vi "Actor Core.vi"(8 "error in":errorcluster, 11 "IViewable In":refnum<class "IViewable.lvclass">) -> (0 "error out":errorcluster, 3 "Actor out":refnum<class "Actor.lvclass">)   [LabVIEW 2017, in "IViewable.lvlib" / "IViewable.lvclass"]
doc: "(<B>Filename</B>: Actor Framework.lvlib:Actor.lvclass:Actor Core.vi)\n\nReceives messages to the actor, reacts to them, and initiates any error handling that may shut the actor down.\n\nDescendant classes may override this VI to append parallel tasks for the actor to complete while it handles messages. Overrides use the Call Parent Method node.\n\n<License>\nCopyright © 2017 Composed Systems, LLC | All rights reserved\nwww.composed.io\n\nAuthor: Ethan Stern <ethan.stern@composed.io>\n\nThis software is provided \"AS IS\" WITHOUT WARRANTIES, either express or implied, AND IS FOR EDUCATIONAL PURPOSES ONLY.\n</License>"
uses:
  IViewable.lvclass
  C:/Program Files (x86)/National Instruments/LabVIEW 2017/vi.lib/ActorFramework/Actor/Actor.lvclass
  <vilib>/ActorFramework/Actor/Actor.lvclass
  IViewable.lvclass/IViewable.ctl
  <vilib>/ActorFramework/Actor/Actor.lvclass/Actor.ctl
  <vilib>/ActorFramework/Message Enqueuer/Message Enqueuer.lvclass/Message Enqueuer.ctl
  IViewable Messages/Resize Panel to Pane Msg/Resize Panel to Pane Msg.lvclass/Resize Panel to Pane Msg.ctl
  <vilib>/ActorFramework/Message Enqueuer/Init from Existing Queue.vi
  <vilib>/ActorFramework/Message Enqueuer/Enqueue.vi
  IViewable Messages/Resize Panel to Pane Msg/Resize Panel to Pane Msg.lvclass
  C:/Program Files (x86)/National Instruments/LabVIEW 2017/vi.lib/ActorFramework/Message/Message.lvclass
  <vilib>/ActorFramework/Message Priority Queue/Priority Enqueue.vi
  <vilib>/ActorFramework/Message Enqueuer/Message Enqueuer.lvclass
  ActorEvents/IEventAggregator/IEventAggregator.lvclass
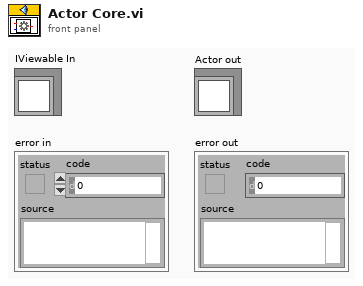
[diagram p1: front panel]
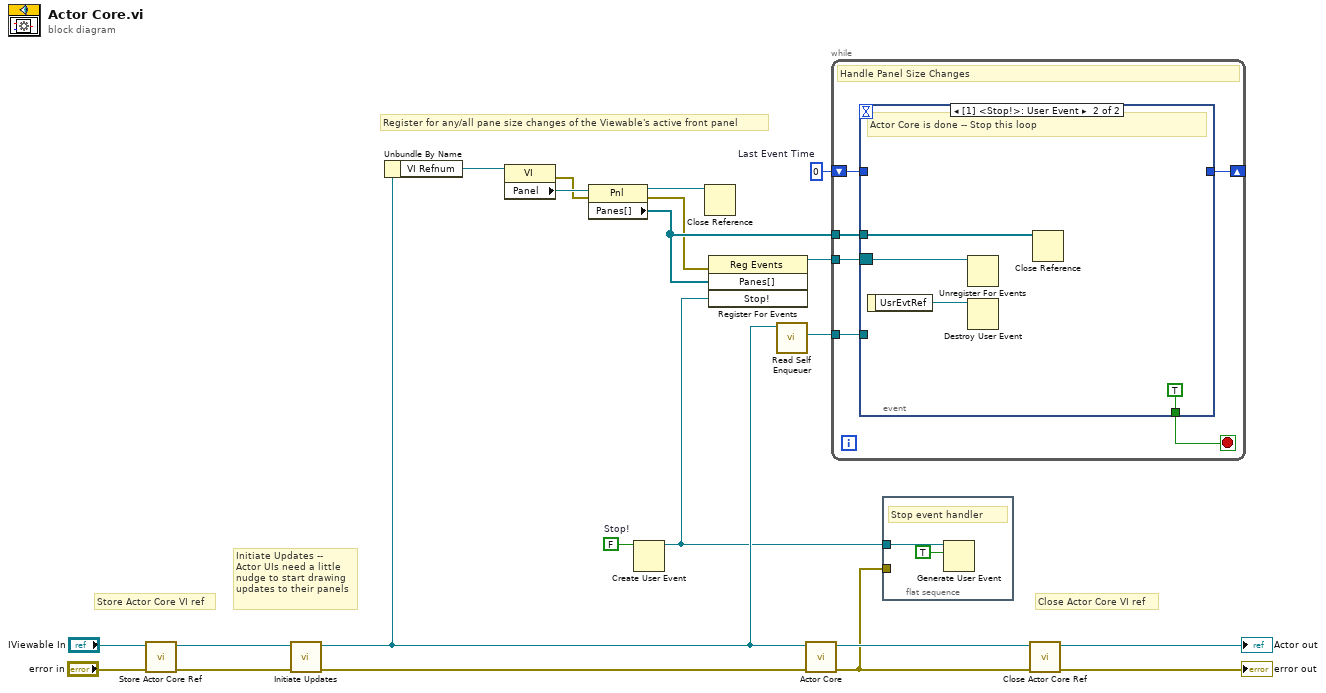
[diagram p0: block diagram]
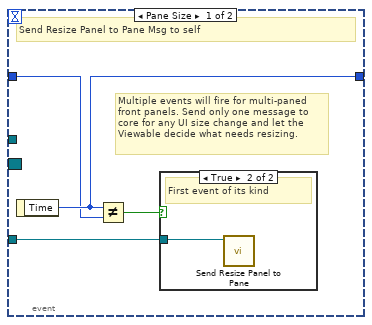
[diagram p2: hidden frame]
diagram:
  w4 = u32 0  # Last Event Time
  w8 = FALSE  # Stop!
  # "Close Actor Core VI ref"
  # "Register for any/all pane size changes of the Viewable's active front panel"
  # "Initiate Updates --\nActor UIs need a little\nnudge to start drawing\nupdates to their panels"
  # "Store Actor Core VI ref"
  n1 = call "Store Actor Core Ref.vi"("error in (no error)"="error in", "IViewable In"="IViewable In") -> ("error out"=w15:errorcluster, "IViewable Out"=w14:refnum<class "IViewable.lvclass">)  [unwired: 8 in]
  n2 = call-dynamic "Initiate Updates.vi"("error in (no error)"=w15, "IViewable In"=w14) -> ("error out"=w6:errorcluster, "IViewable Out"=w13:refnum<class "IViewable.lvclass">)  [unwired: 8 in]
  n3 = Unbundle By Name(w13) -> ("VI Refnum"=w9:refnum<vi>)
  n4 = property class="VI"(reference=w9) -> (error out=w11:errorcluster, "Panel"=w12:refnum<vi>)  [unwired: 1 in, 1 out]
  n5 = property class="Pnl"(reference=w12, error in=w11) -> (reference out=w5:refnum<vi>, error out=w10:errorcluster, "Panes[]"=w16:refnum<vi>[])
  n6 = Create User Event(user event datatype=w8) -> (user event=w7:refnum<user-event>)  [unwired: 1 in, 1 out]
  n7 = Close Reference(reference=w5) -> ()  [unwired: 1 in, 1 out]
  n8 = register-events(error in=w10, w16, w7) -> (reference out=w18:refnum<event-registration>)  [unwired: 1 in, 1 out]
  n9 = call <vilib>:"Read Self Enqueuer.vi"("Actor"=w13) -> ("Self Enqueuer"=w17:refnum<class "Message Enqueuer.lvclass">)  [unwired: 10 in]
  n10 = call-parent "Actor Core.vi"("error in"=w6, "Actor in"=w13) -> ("error out"=w2:errorcluster, "Actor out"=w19:refnum<class "Actor.lvclass">)  [unwired: 8 in]
  n11 = while {
    tunnel: w18 -> [w27]
    tunnel: w17 -> [w26]
    tunnel: w16 -> [w24]
    shift-right: [w23] -> _
    shift-left: w4 -> [w22]
    stop <- w25 stop-if-true
    # "Handle Panel Size Changes"
    n12 = event shown="[1] <Stop!>: User Event" {
      selector: w27 -> [_ w34]
      dyn-events: _ -> [_ _]
      timeout: _ -> [_ _]
      tunnel: w26 -> [w28 _]
      tunnel: [_ TRUE] -> w25
      tunnel: w24 -> [_ w35]
      tunnel: [w31 _] -> w23
      tunnel: w22 -> [w30 _]
      event Pane Size {
        # "Multiple events will fire for multi-paned\nfront panels. Send only one message to\ncore for any UI size change and let the\nViewable decide what needs resizing."
        # "Send Resize Panel to Pane Msg to self"
        n13 = event-data() -> ("Time"=w31:u32)  [unwired: 1 in]
        n14 = Not Equal?(x=w31, y=w30) -> (x != y?=w29:bool)
        n15 = case shown="True" w29 {
          tunnel: w28 -> [_ w32]
          frame False {
            # "Flush redundant events"
          }
          frame True {
            # "First event of its kind"
            n16 = call "Send Resize Panel to Pane.vi"("Message Enqueuer"=w32) -> ()  [unwired: 9 in, 2 out]
          }
        }
      }
      event User Event {
        # "Actor Core is done -- Stop this loop"
        n17 = event-data() -> ("UsrEvtRef"=w33:refnum<user-event>)  [unwired: 1 in]
        n18 = Unregister For Events(event registration refnum=w34) -> ()  [unwired: 1 in, 1 out]
        n19 = Destroy User Event(user event=w33) -> ()  [unwired: 1 in, 1 out]
        n20 = Close Reference(reference=w35) -> ()  [unwired: 1 in, 1 out]
      }
    }
  }
  n21 = flat-sequence {
    tunnel: w2 -> [_]
    tunnel: w7 -> [w38]
    frame #0 {
      # "Stop event handler"
      n22 = Generate User Event(user event=w38, event data cluster=TRUE) -> ()  [unwired: 2 in, 2 out]
    }
  }
  n23 = call "Close Actor Core Ref.vi"("error in (no error)"=w2, "Actor in"=w19) -> ("error out"=→"error out":errorcluster, "Actor out"=→"Actor out":refnum<class "Actor.lvclass">)  [unwired: 8 in]
